vi "Conditional Add 1 [I32].vi"(1 "Condition":bool=TRUE, 2 "x":i32) -> (7 "x (+1)":i32)   [LabVIEW 2021]
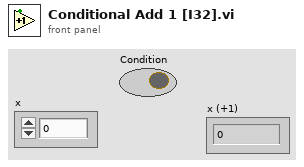
[diagram p1: front panel]
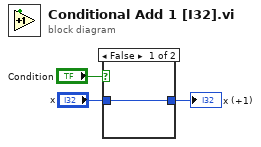
[diagram p0: block diagram]
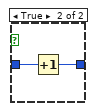
[diagram p2: hidden frame]
diagram:
  n1 = case shown="False" "Condition" {
    tunnel: [w4 w6] -> w3
    tunnel: "x" -> [w4 w5]
    frame False {
    }
    frame True {
      n2 = Increment(x=w5) -> (x+1=w6:i32)
    }
  }
  "x (+1)" <- w3
